vi "Init Close eFGV.vi"(6 "State":T1, 8 "error in (no error)":errorcluster) -> (0 "error out":errorcluster)   [LabVIEW 2020]
uses:
  Shared/Control/State - eFGV.ctl
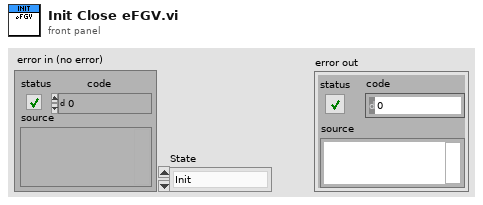
[diagram p1: front panel]
types:
  T1 = typedef "State - eFGV.ctl" = enum16{"Init", "Read", "Write", "Close"}
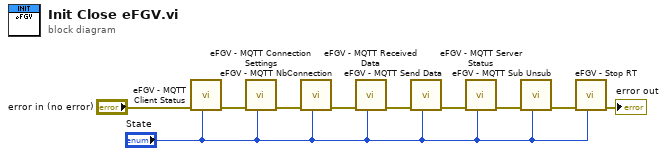
[diagram p0: block diagram]
diagram:
  n1 = call "eFGV - MQTT Client Status.vi"("State"="State", "error in (no error)"="error in (no error)") -> ("error out"=w8:errorcluster)  [unwired: 8 in, 1 out]
  n2 = call "eFGV - MQTT Connection Settings.vi"("State"="State", "error in (no error)"=w8) -> ("error out"=w7:errorcluster)  [unwired: 8 in, 1 out]
  n3 = call "eFGV - MQTT NbConnection.vi"("State"="State", "error in (no error)"=w7) -> ("error out"=w6:errorcluster)  [unwired: 8 in, 1 out]
  n4 = call "eFGV - MQTT Received Data.vi"("State"="State", "error in (no error)"=w6) -> ("error out"=w5:errorcluster)  [unwired: 8 in, 1 out]
  n5 = call "eFGV - MQTT Send Data.vi"("State"="State", "error in (no error)"=w5) -> ("error out"=w4:errorcluster)  [unwired: 8 in, 1 out]
  n6 = call "eFGV - MQTT Server Status.vi"("State"="State", "error in (no error)"=w4) -> ("error out"=w3:errorcluster)  [unwired: 8 in, 1 out]
  n7 = call "eFGV - MQTT Sub Unsub.vi"("State"="State", "error in (no error)"=w3) -> ("error out"=w2:errorcluster)  [unwired: 8 in, 1 out]
  n8 = call "eFGV - Stop RT.vi"("State"="State", "error in (no error)"=w2) -> ("error out"=→"error out":errorcluster)  [unwired: 8 in, 1 out]
